vi "create context.vi"(8 "error in (no error)":errorcluster, 11 "Socket in":refnum<class "Socket.lvclass">) -> (0 "error out":errorcluster, 3 "Socket out":refnum<class "Socket.lvclass">)   [LabVIEW 2018, in "Socket.lvclass"]
uses:
  Socket.lvclass
  Socket.lvclass/Socket.ctl
  <vilib>/addons/zeromq/zmq_context.lvclass
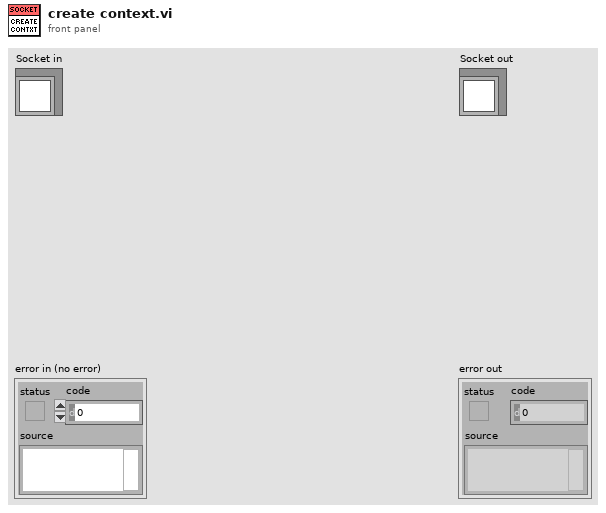
[diagram p1: front panel]
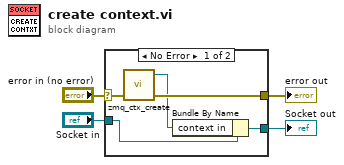
[diagram p0: block diagram]
diagram:
  n1 = case shown="No Error" "error in (no error)" {
    selector: "error in (no error)" -> [w9 w11]
    tunnel: [w8 w11] -> w3
    tunnel: [w6 w10] -> w1
    tunnel: "Socket in" -> [w7 w10]
    frame No Error {
      n2 = call <vilib>:"zmq_ctx_create.vi"("error in"=w9) -> ("error out"=w8:errorcluster, "context out"=w5:refnum<class "zmq_context.lvclass">)  [unwired: 3 in]
      n3 = Bundle By Name(cluster=w7, "context in"=w5) -> (w6:refnum<class "Socket.lvclass">)
    }
    frame Error {
    }
  }
  "error out" <- w3
  "Socket out" <- w1
